vi "make 2d scan file with multibin drift check.vi"() -> ()   [LabVIEW 2013]
uses:
  scan parameters.ctl
panel:
  in  "Multibin":i16
  in  "check value":dbl=0.00012914
  in  "start scan":i32
  in  "precision (12)":i16=12
  in  "reverse which par is scanned":bool
  in  "2D scan details":T2(array[cluster])=[{"Scan parameters"={"Scan Start"=1.1e-06, "Scan End"=2.1e-06, "Scan Step Size"=5e-08, "# Shots Each Step"=7, "single direction?"=TRUE}, "device and variable preamble"="Device = \"HeatHighlandT564\"\nVariable = \"Discharge timing s\""}, {"Scan parameters"={"Scan Start"=10.0, "Scan End"=70.0, "Scan Step Size"=5.0, "# Shots Each Step"=1, "single direction?"=TRUE}, "device and variable preamble"="Device = \"PL1-PresCtrl-Low1\"\nVariable = \"P. Control Down (Torr)\""}] {"Scan parameters"."Scan Start" format="%#.9p"; "Scan parameters"."Scan End" format="%#.9p"; "Scan parameters"."Scan Step Size" format="%#.9p"}
  out "spreadsheet string":string
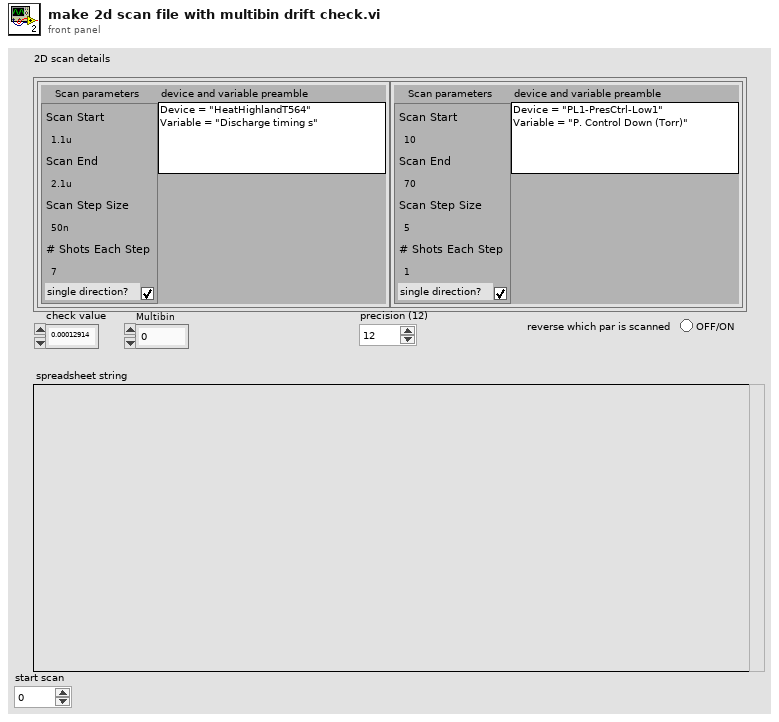
[diagram p1: front panel]
types:
  T1 = typedef "scan parameters.ctl" = cluster{"Scan Start":dbl, "Scan End":dbl, "Scan Step Size":dbl, "# Shots Each Step":u32, "single direction?":bool}
  T2 = cluster{"Scan parameters":T1, "device and variable preamble":string}[]
  T3 = cluster{"Scan parameters":T1, "device and variable preamble":string}
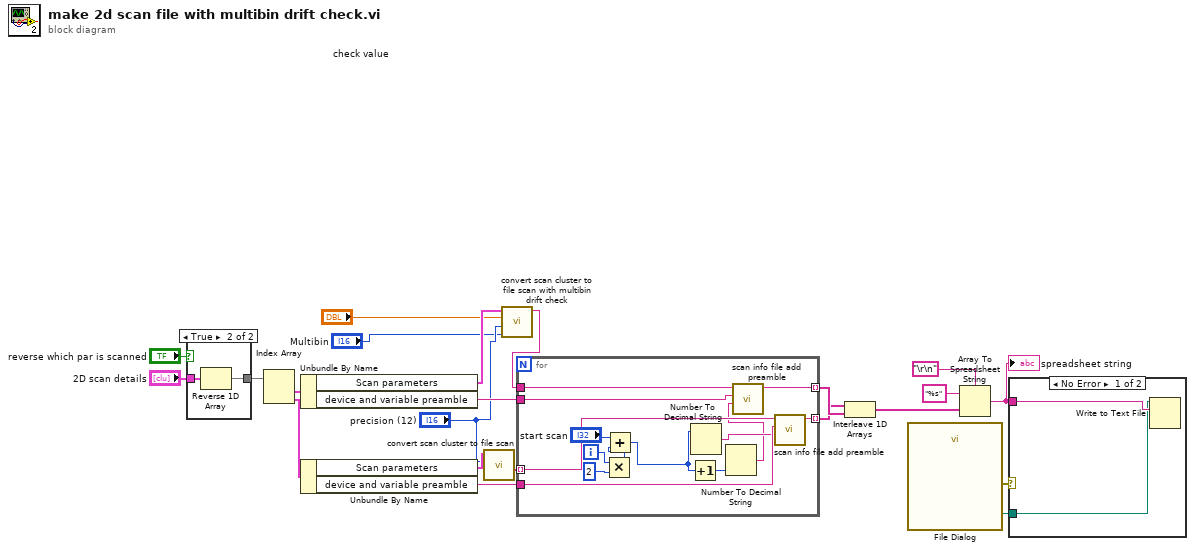
[diagram p0: block diagram]
diagram:
  n1 = case shown="True" "reverse which par is scanned" {
    tunnel: "2D scan details" -> [w23 w25]
    tunnel: [w23 w24] -> w11
    frame False {
    }
    frame True {
      n2 = Reverse 1D Array(array=w25) -> (reversed array=w24:T2)
    }
  }
  n3 = Index Array(array=w11) -> (element #1=w9:T3, element #2=w8:T3)  [unwired: 2 in]
  n4 = Unbundle By Name(w9) -> ("Scan parameters"=w5:T1, "device and variable preamble"=w13:string)
  n5 = Unbundle By Name(w8) -> ("Scan parameters"=w7:T1, "device and variable preamble"=w6:string)
  n6 = call "convert scan cluster to file scan.vi"("precision (12)"="precision (12)", "Scan parameters"=w7) -> ("values:numshots"=w19:string[])  [unwired: 7 in, 2 out]
  n7 = call "convert scan cluster to file scan with multibin drift check.vi"("Scan parameters"=w5, "check value"="check value", "precision (12)"="precision (12)", "multibin"="Multibin") -> ("spreadsheet string"=w2:string)  [unwired: 4 in, 2 out]
  n8 = for {
    tunnel: [w37] -> w20 mode=indexing
    tunnel: w2 -> [w38]
    tunnel: w19 -> [w35] mode=indexing
    tunnel: [w34] -> w17 mode=indexing
    tunnel: w13 -> [w33]
    tunnel: w6 -> [w32]
    i -> [w29]
    n9 = Multiply(x=w29, y=2) -> (x*y=w28:i32)
    n10 = Add(x="start scan", y=w28) -> (x+y=w26:i32)
    n11 = Increment(x=w26) -> (x+1=w36:i32)
    n12 = Number To Decimal String(number=w26) -> (decimal integer string=w31:string)  [unwired: 1 in]
    n13 = Number To Decimal String(number=w36) -> (decimal integer string=w30:string)  [unwired: 1 in]
    n14 = call "scan info file add preamble.vi"("scan #"=w30, "device and variable stuff"=w33, "spreadsheet string"=w38) -> ("scan text for txt file"=w37:string)  [unwired: 8 in]
    n15 = call "scan info file add preamble.vi"("scan #"=w31, "device and variable stuff"=w32, "spreadsheet string"=w35) -> ("scan text for txt file"=w34:string)  [unwired: 8 in]
  }
  n16 = Interleave 1D Arrays(w17, w20) -> (w18:string[])
  n17 = call "File Dialog"() -> ("selected path"=w14:path, "error out"=w15:errorcluster)  [unwired: 12 in, 2 out]
  n18 = Array To Spreadsheet String(delimiter (Tab)="\r\n", array=w18, 3:"%s" ("format string")) -> (spreadsheet string=w16:string)
  "spreadsheet string" <- w16
  n19 = case shown="No Error" w15 {
    tunnel: w16 -> [w41 _]
    tunnel: w14 -> [w40 _]
    frame No Error {
      n20 = Write to Text File(file (use dialog)=w40, text=w41) -> ()  [unwired: 2 in, 3 out]
    }
    frame Error {
    }
  }
